vi "plot2.vi"(8 "error in (no error)":errorcluster, 11 "Counter in":refnum<class "Counter.lvclass">) -> (0 "error out":errorcluster, 3 "Counter out":refnum<class "Counter.lvclass">)   [LabVIEW 2013, in "Counter.lvclass"]
uses:
  Counter.lvclass
  Counter.lvclass/Counter.ctl
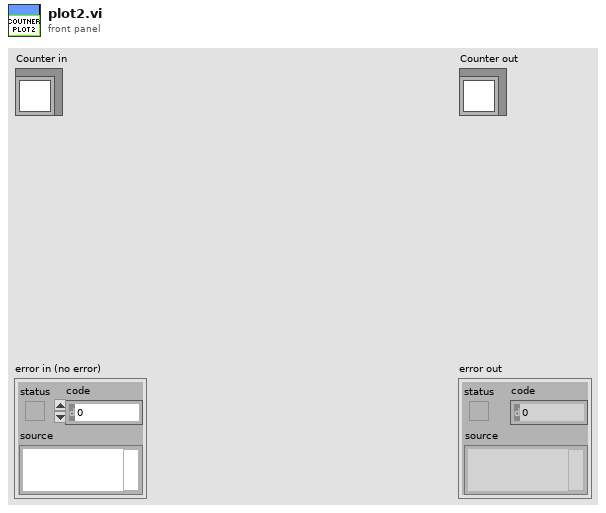
[diagram p1: front panel]
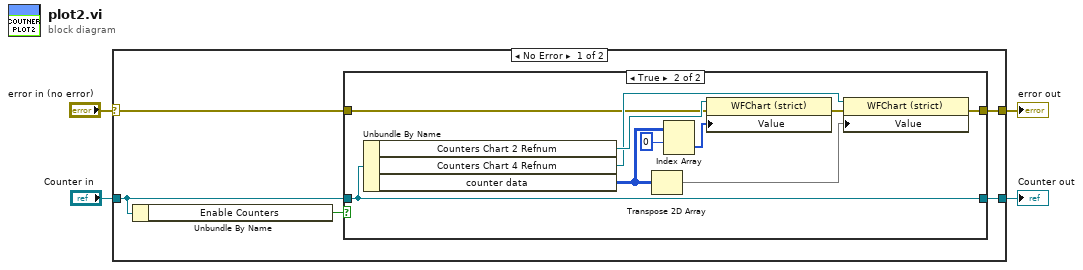
[diagram p0: block diagram]
diagram:
  n1 = case shown="No Error" "error in (no error)" {
    selector: "error in (no error)" -> [w9 w23]
    tunnel: [w8 w23] -> w3
    tunnel: [w7 w22] -> w1
    tunnel: "Counter in" -> [w6 w22]
    frame No Error {
      n2 = Unbundle By Name(w6) -> ("Enable Counters"=w5:bool)
      n3 = case shown="True" w5 {
        tunnel: w9 -> [w11 w15]
        tunnel: [w11 w14] -> w8
        tunnel: w6 -> [w10 w12]
        tunnel: [w10 w12] -> w7
        frame False {
        }
        frame True {
          n4 = Unbundle By Name(w12) -> ("Counters Chart 2 Refnum"=w21:refnum<vi>, "Counters Chart 4 Refnum"=w20:refnum<vi>, "counter data"=w13:u32[][])
          n5 = Transpose 2D Array(2D array=w13) -> (transposed array=w17:u32[][])
          n6 = Index Array(array=w13, index (row)=0) -> (element=w18:u32[])  [unwired: 1 in]
          n7 = property class="WFChart (strict)"(reference=w21, error in=w15, "Value"=w18) -> (error out=w19:errorcluster)  [unwired: 1 out]
          n8 = property class="WFChart (strict)"(reference=w20, error in=w19, "Value"=w17) -> (error out=w14:errorcluster)  [unwired: 1 out]
        }
      }
    }
    frame Error {
    }
  }
  "error out" <- w3
  "Counter out" <- w1
